vi "Credit Update.vi"(8 "error in (no error)":errorcluster, 10 "Credit":dbl, 11 "UI Actor in":refnum<class "UI Actor.lvclass">) -> (0 "error out":errorcluster, 3 "UI Actor out":refnum<class "UI Actor.lvclass">)   [LabVIEW 2020, in "UI Actor.lvlib" / "UI Actor.lvclass"]
uses:
  UI Actor.lvclass
  UI Actor.lvclass/UI Actor.ctl
  Messages Actor Messages/Update message Msg/Update message Msg.lvclass/Update message Msg.ctl
  <vilib>/ActorFramework/Message Enqueuer/Message Enqueuer.lvclass/Message Enqueuer.ctl
  <vilib>/ActorFramework/Message Enqueuer/Enqueue.vi
  Messages Actor Messages/Update message Msg/Update message Msg.lvclass
  C:/Program Files (x86)/National Instruments/LabVIEW 2020/vi.lib/ActorFramework/Message/Message.lvclass
  <vilib>/ActorFramework/Message Priority Queue/Priority Enqueue.vi
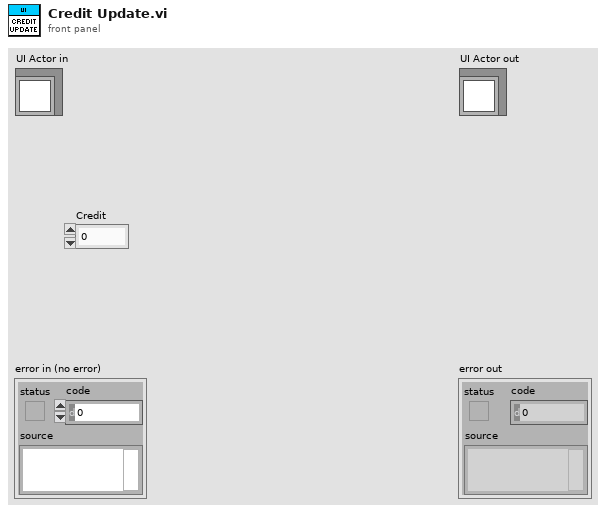
[diagram p1: front panel]
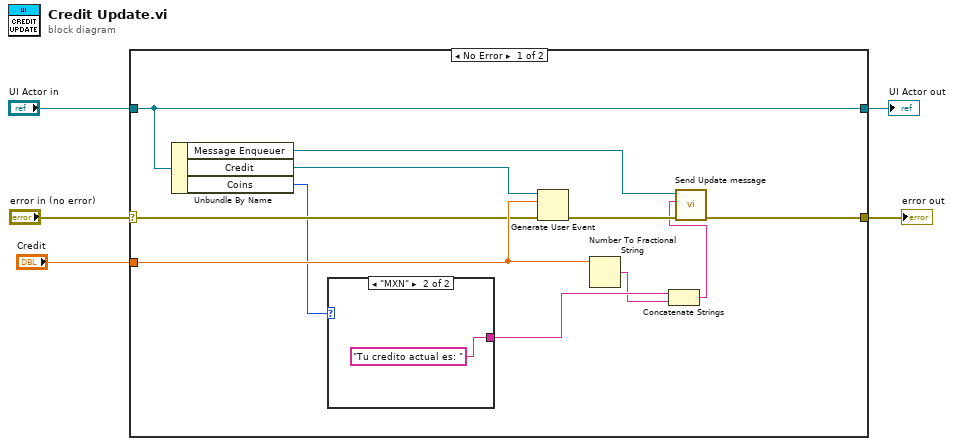
[diagram p0: block diagram]
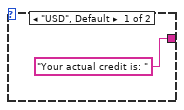
[diagram p2: hidden frame]
diagram:
  n1 = case shown="No Error" "error in (no error)" {
    selector: "error in (no error)" -> [w11 w20]
    tunnel: [w10 w20] -> w4
    tunnel: [w15 w19] -> w2
    tunnel: "UI Actor in" -> [w15 w19]
    tunnel: "Credit" -> [w14 _]
    frame No Error {
      n2 = Unbundle By Name(w15) -> ("Message Enqueuer"=w12:refnum<class "Message Enqueuer.lvclass">, "Credit"=w16:refnum<user-event>, "Coins"=w9:enum16{"USD", "MXN"})
      n3 = case shown="\"MXN\"" w9 {
        tunnel: ["Your actual credit is: " ("message") "Tu credito actual es: " ("message")] -> w8
        frame "USD", Default {
        }
        frame "MXN" {
        }
      }
      n4 = Generate User Event(user event=w16, event data cluster=w14, error in=w11) -> (error out=w13:errorcluster)  [unwired: 1 in, 1 out]
      n5 = Number To Fractional String(number=w14) -> (F-format string=w7:string)  [unwired: 3 in]
      n6 = Concatenate Strings(w8, w7) -> (w6:string)
      n7 = call "Send Update message.vi"("error in (no error)"=w13, "Update msg"=w6, "Message Enqueuer"=w12) -> ("error out"=w10:errorcluster)  [unwired: 7 in, 1 out]
    }
    frame Error {
    }
  }
  "error out" <- w4
  "UI Actor out" <- w2
